vi "Create.vi"(8 "error in (no error)":errorcluster, 10 "Input":string) -> (0 "error out":errorcluster, 3 "Network":refnum<class "Stateless Network.lvclass">)   [LabVIEW 2020, in "Stateless Network.lvclass"]
uses:
  Stateless Network.lvclass
  Stateless Network.lvclass/Stateless Network.ctl
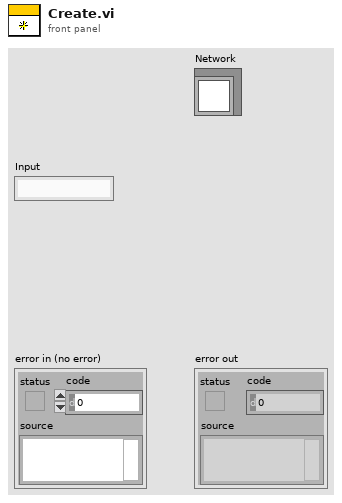
[diagram p1: front panel]
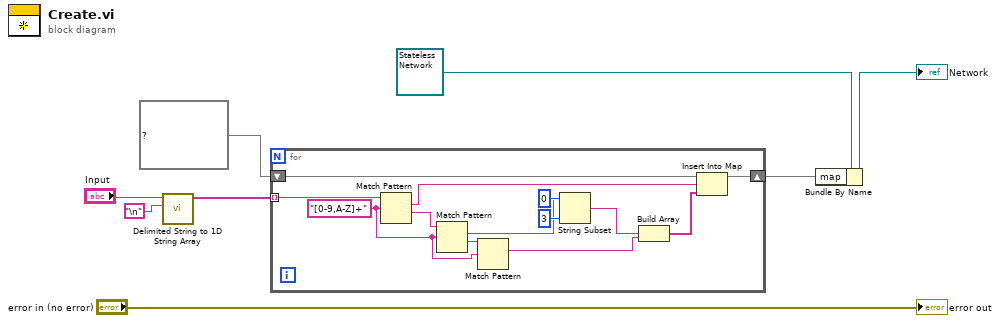
[diagram p0: block diagram]
diagram:
  n1 = call <vilib>:"Delimited String to 1D String Array.vi"("delimiter"="\n", "delimited string"="Input") -> ("string array"=w4:string[])  [unwired: 9 in]
  n2 = for {
    tunnel: w4 -> [w21] mode=indexing
    shift-right: [w16] -> w1
    shift-left: map{string, string[]} {} ("map") -> [w17]
    w13 = "[0-9,A-Z]+" ("regular expression")
    n3 = Match Pattern(string=w21, regular expression=w13) -> (match substring=w15:string, after substring=w20:string)  [unwired: 1 in, 2 out]
    n4 = Match Pattern(string=w20, regular expression=w13) -> (match substring=w10:string, after substring=w19:string)  [unwired: 1 in, 2 out]
    n5 = Match Pattern(string=w19, regular expression=w13) -> (match substring=w18:string)  [unwired: 1 in, 3 out]
    n6 = String Subset(string=w10, offset (0)=0, length (rest)=3 ("length (rest)")) -> (substring=w9:string)
    n7 = Build Array(w9, w18) -> (w14:string[])
    n8 = Insert Into Map(map in=w17, key=w15, value=w14) -> (map out=w16:map{string, string[]})  [unwired: 2 out]
  }
  n9 = Bundle By Name(cluster=refnum<class "Stateless Network.lvclass"> refnum ("Network"), "map"=w1) -> (→"Network":refnum<class "Stateless Network.lvclass">)
  "error out" <- "error in (no error)"
